vi "data_rate.vi"(1 "GPIB address":string) -> (0 "Data rate (Hz)":dbl format="%.1f")   [LabVIEW 2010]
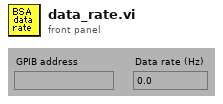
[diagram p1: front panel]
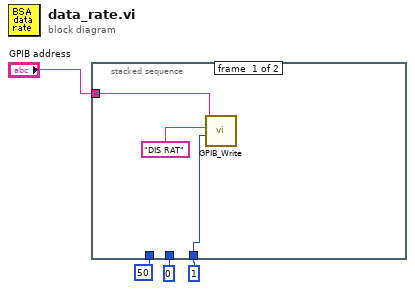
[diagram p0: block diagram]
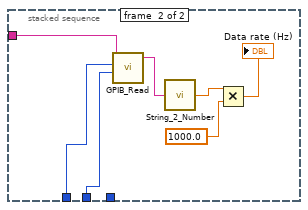
[diagram p2: hidden frame]
diagram:
  n1 = stacked-sequence {
    tunnel: "GPIB address" -> [w7 w14]
    tunnel: 1 -> [w5 _]
    tunnel: 0 -> [_ w13]
    tunnel: 50 -> [_ w12]
    frame #0 {
      n2 = call "GPIB_Write.vi"("address string"=w7, "data In"="DIS RAT", "mode (0)"=w5) -> ()  [unwired: 2 in, 2 out]
    }
    frame #1 {
      n3 = call "GPIB_Read.vi"("address string"=w14, "byte count"=w12, "mode (0)"=w13) -> ("data Out"=w11:string)  [unwired: 2 in, 2 out]
      n4 = call "String_2_Number.vi"("Value"=w11) -> ("Numeric"=w8:dbl)
      n5 = Multiply(x=w8, y=1000.0) -> (x*y=→"Data rate (Hz)":dbl)
    }
  }
